vi "FTW-CodeGen-Prototype.vi"(0 "ADAPT_Type and Defaults":cluster{"Element":variant}, 5 "REPLACED_JSON String":string, 11 "REPLACED_error in":errorcluster) -> (4 "ADAPT_Values":cluster{"Element":variant}, 15 "REPLACED_error out":errorcluster)   [LabVIEW 2013, in "FTW-JSON-Deserialize.xnode"]
uses:
  FTW-JSON-Deserialize.xnode
  Error/FTW-ERR-NoErrorConstant.vi
  Error/FTW-ERR-ThrowError.vi
  Error/FTW-ERR-ThrowGenericError.vi
panel:
  # "Inputs"
  # "Outputs"
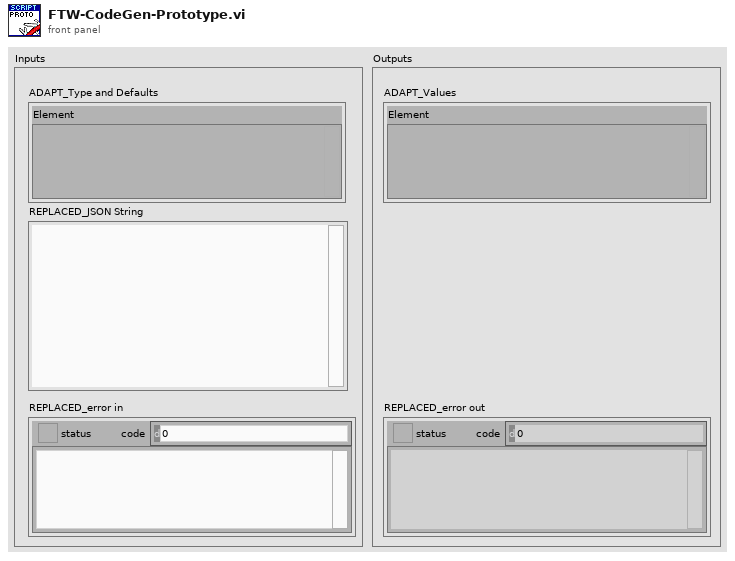
[diagram p1: front panel]
types:
  T1 = typedef "FTW-Reflection-Types.ctl" = enum16{"Unknown", "Void", "Array", "Cluster", "LVObject", "Boolean", "I8", "I16", "I32", "I64", "U8", "U16", "U32", "U64", "SGL", "DBL", "EXT", "CSG", "CDB", "CXT", "FXP", "EnumU8", "EnumU16", "EnumU32", "EnumU64", "SGLwithUnit", "DBLwithUnit", "EXTwithUnit", "CSGwithUnit", "CDBwithUnit", "CXTwithUnit", "String", "Path", "Picture", "Tag", "LVVariant", "Timestamp", "WaveformI8", "WaveformI16", "WaveformI32", "WaveformI64", "WaveformU8", "WaveformU16", "WaveformU32", "WaveformU64", "WaveformSGL", "WaveformDBL", "WaveformEXT", "WaveformCSG", "WaveformCDB", "WaveformCXT", "WaveformDigital", "WaveformUnknownType", "DigitalData", "DynamicData", "ExternalData", "FileByteStream", "TDMStream", "dotNET", "ActiveX", "VIServerReference", "VIReference", "ApplicationInstance", "Menu", "ConnectionDataSocket", "ConnectionVISA", "ConnectionBluetooth", "ConnectionIrDA", "ConnectionTCP", "ConnectionUDP", "ConnectionHTTPClient", "ConnectionFTP", "Occurrence", "Notifier", "Queue", "Rendezvous", "Semaphore", "RTFIFO", "EventPublisher", "EventRegistration", "EventCallback", "DataValueReference", "GenericClass", "GenericClassTag", "GenericClassDeepCopy", "GenericClassFlattened", "GenericClassTagFlattened", "GenericReferenceType", "WindowsRegistry", "OverloadedDatalogRef", "ReferenceUnknownType"}
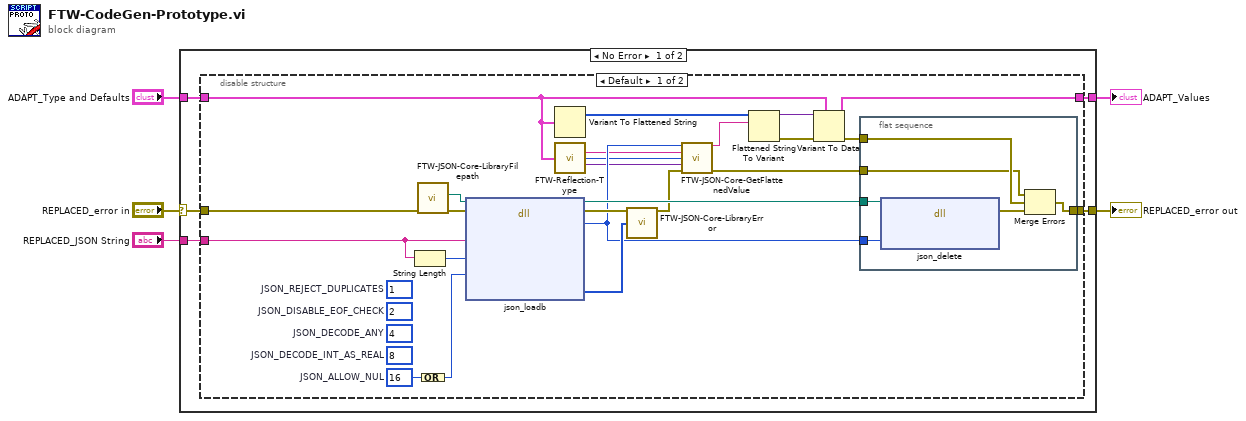
[diagram p0: block diagram]
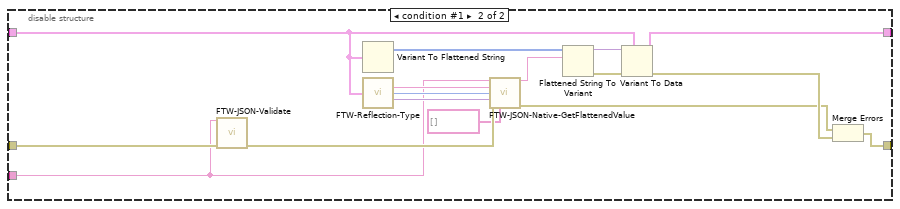
[diagram p2: hidden frame]
diagram:
  n1 = case shown="No Error" "REPLACED_error in" {
    selector: "REPLACED_error in" -> [w8 w58]
    tunnel: "REPLACED_JSON String" -> [w7 _]
    tunnel: [w6 w58] -> w1
    tunnel: "ADAPT_Type and Defaults" -> [w10 w57]
    tunnel: [w9 w57] -> w3
    frame No Error {
      n2 = disable-structure shown="Default" {
        disable-tunnel: w10 -> [w14 w44]
        disable-tunnel: [w34 w56] -> w9
        disable-tunnel: w8 -> [w26 w55]
        disable-tunnel: w7 -> [w25 w46]
        disable-tunnel: [w20 w53] -> w6
        frame condition #0 (active) {
          w27 = u64 16  # JSON_ALLOW_NUL
          (unwired) u64 8  # JSON_DECODE_INT_AS_REAL
          (unwired) u64 4  # JSON_DECODE_ANY
          (unwired) u64 2  # JSON_DISABLE_EOF_CHECK
          (unwired) u64 1  # JSON_REJECT_DUPLICATES
          n3 = String Length(string=w25) -> (length=w29:i32)
          n4 = call "FTW-JSON-Core-LibraryFilepath.vi"("error in"=w26) -> ("error out"=w33:errorcluster, "JSON Library Filepath"=w32:path)  [unwired: 9 in]
          n5 = Compound Arithmetic op=OR(w27) -> (w28:u64)
          n6 = dll-call lib="?" fn="json_loadb"(path in=w32, error in=w33, "JSON Buffer"=w25, "Buffer Size"=w29, "Flags"=w28) -> (path out=w24:path, error out=w31:errorcluster, "JSON Object Pointer"=w22:i64, "Error Structure"=w30:u8[])  [unwired: 5 in]
          n7 = Variant To Flattened String(Variant=w14) -> (1:w11:i16[])  [unwired: 1 out]
          n8 = call "FTW-Reflection-Type.vi"("Anything"=w14) -> ("Data Name"=w17:string, "LabVIEW Type"=w16:T1, "Variant Type and Value"=w15:variant)  [unwired: 12 in]
          n9 = call "FTW-JSON-Core-LibraryError.vi"("error in"=w31, "Error Structure"=w30) -> ("error out"=w23:errorcluster)  [unwired: 13 in]
          n10 = call "FTW-JSON-Core-GetFlattenedValue.vi"("JSON Element"=w22, "Element Data Name"=w17, "LabVIEW Type"=w16, "Element Default Value"=w15, "error in"=w23) -> ("Flattened Value"=w19:string, "error out"=w18:errorcluster)  [unwired: 9 in]
          n11 = Flattened String To Variant(6:w19, 7:w11) -> (0:w13:errorcluster, 3:w12:variant)  [unwired: 1 in]
          n12 = Variant To Data(error in=w13, type=w14, Variant=w12) -> (data=w34:cluster{"Element":variant}, error out=w21:errorcluster)
          n13 = flat-sequence {
            tunnel: w24 -> [w40]
            tunnel: w22 -> [w39]
            tunnel: w21 -> [w38]
            tunnel: [w36] -> w20
            tunnel: w18 -> [w35]
            frame #0 {
              n14 = dll-call lib="?" fn="json_delete"(path in=w40, "JSON Object Pointer"=w39) -> (error out=w37:errorcluster)  [unwired: 4 in, 1 out]
              n15 = Merge Errors(w35, w38, w37) -> (w36:errorcluster)
            }
          }
        }
        frame condition #1 {
          n16 = call "FTW-JSON-Validate.vi"("JSON Opject"=w46, "error in"=w55) -> ("error out"=w47:errorcluster)  [unwired: 13 in]
          n17 = Variant To Flattened String(Variant=w44) -> (1:w41:i16[])  [unwired: 1 out]
          n18 = call "FTW-Reflection-Type.vi"("Anything"=w44) -> ("Data Name"=w50:string, "LabVIEW Type"=w49:T1, "Variant Type and Value"=w48:variant)  [unwired: 12 in]
          n19 = call "FTW-JSON-Native-GetFlattenedValue.vi"("JSON String"=w46, "Element Data Name"=w50, "LabVIEW Type"=w49, "Element Default Value"=w48, "error in"=w47, "Pointer"=string[] []) -> ("Flattened Value"=w52:string, "error out"=w51:errorcluster)  [unwired: 8 in]
          n20 = Flattened String To Variant(6:w52, 7:w41) -> (0:w42:errorcluster, 3:w43:variant)  [unwired: 1 in]
          n21 = Variant To Data(error in=w42, type=w44, Variant=w43) -> (data=w56:cluster{"Element":variant}, error out=w54:errorcluster)
          n22 = Merge Errors(w51, w54) -> (w53:errorcluster)
        }
      }
    }
    frame Error {
    }
  }
  "REPLACED_error out" <- w1
  "ADAPT_Values" <- w3
